vi "Updater Version Check.vi"(8 "에러 입력":errorcluster caption="에러 입력(에러 없음)") -> (0 "에러 출력":errorcluster, 1 "서버버전":string, 3 "업데이트?":bool)   [LabVIEW 2020]
uses:
  Support/Controls/Cmd_File path.ctl
  Support/Controls/Cmd_File Type.ctl
  Support/Controls/Cmd_Read Query.ctl
  Support/Public/Polymorph/ini Ctrl_Str.vi
  <vilib>/Utility/config.llb/Read Key (String).vi
  <vilib>/Utility/config.llb/NI_LVConfig.lvlib
  <vilib>/addons/database/NI_Database_API.lvlib
panel:
  out "로컬버전":string caption="값"
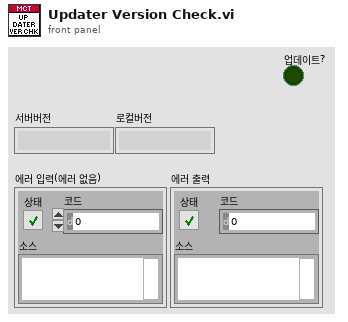
[diagram p1: front panel]
types:
  T1 = typedef "Cmd_Read Query.ctl" = enum16{"교정자 이름 얻기", "인증교정자 얻기", "기술책임자 얻기", "기책부책 얻기", "등록번호 얻기", "등록정보 얻기", "업체정보 얻기", "교정일자(CAMAS) 얻기", "교정일자(CALSTD) 얻기", "교정환경 얻기", "교정절차서 목록 얻기", "교정절차서명 얻기", "교정절차 목록얻기", "교정절차 얻기", "PROC 교정절차 얻기", "PROC SPEC 얻기", "교정절차(Func별) 얻기", "교정절차(Func_ext별) 얻기", "기관코드 얻기", "교정기능(세부분류) 얻기", "교정기능(모델) 얻기", "교정기능 목록 얻기", "교정기능 명칭 얻기", "교정기능 항목명칭 얻기", "DB (사용기준기) 얻기", "DB (기준기이름) 얻기", "DB (기준기이름목록) 얻기", "DB (기준기목록) 얻기", "DB (기준기값) 얻기", "DB (CMC) 얻기", "DB (FUNC) 얻기", "DB (CALNAME) 얻기", "DB (STDNAME) 얻기", "DB (SPEC) 얻기", "모델(항목전체) 얻기", "모델(최대범위) 얻기", "모델(최소범위) 얻기", "모델(최대최소) 얻기", "모델(범위조건) 얻기", "모델(등록요청) 얻기", "모델(형식별) 얻기", "모델(조건별) 얻기", "모델(모델검색) 얻기", "세부분류 목록 얻기", "기준기등록리스트 얻기", "STD Cal Date Check", "DB등록일자 얻기", "적용항목 얻기", "기타정보 얻기", "기준기요청 얻기", "서버버전 얻기"}
  T2 = typedef "Cmd_File Type.ctl" = enum16{"엑셀", "엑셀(2003)", "텍스트", "설정", "2진", "VI", "CSV", "LOG", "폴더"}
  T3 = typedef "Cmd_File path.ctl" = enum16{"에러로그", "데이터파일경로", "성적서원본", "지난성적서", "Data Files", "경로생성", "Updater", "Template", "설정파일경로", "FTP Upload", "Update 경로", "어플리케이션"}
  T4 = typedef "NI_Database_API.lvlib/Conn ObjectReference.ctl" = refnum<k1>
  T5 = typedef "NI_LVConfig.lvlib/Config Data RefNum.ctl" = refnum<k1>
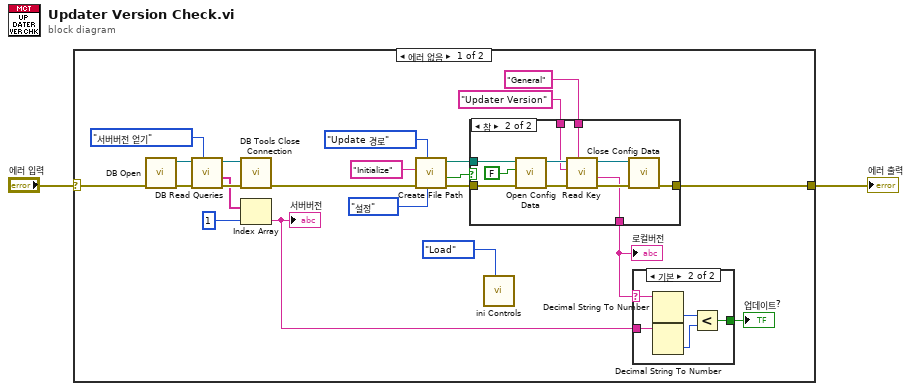
[diagram p0: block diagram]
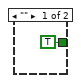
[diagram p2: hidden frame]
diagram:
  n1 = case shown="에러 없음" "에러 입력" {
    selector: "에러 입력" -> [w21 w43]
    tunnel: [w4 w43] -> w2
    frame No Error {
      n2 = call "DB Open.vi"("에러 입력"=w21) -> ("에러 출력"=w10:errorcluster, "참조 번호 출력"=w11:T4)  [unwired: 9 in]
      n3 = call "DB Read Queries.vi"("Query Command"=Cmd_Read_Query."서버버전 얻기", "에러 입력(에러 없음)"=w10, "참조 번호 입력"=w11) -> ("에러 출력"=w8:errorcluster, "Data (0번행)"=w6:string[], "참조 번호 출력"=w9:T4)  [unwired: 4 in, 2 out]
      n4 = call <vilib>:"DB Tools Close Connection.vi"("error in (no error)"=w8, "connection reference"=w9) -> ("error out"=w20:errorcluster)  [unwired: 5 in]
      n5 = Index Array(array=w6, index=1 ("비활성화된 인덱스 (열)")) -> (element=w14:string)
      "서버버전" <- w14
      n6 = call "Create File Path.vi"("파일타입"=Cmd_File_Type."설정", "항목"=Cmd_File_path."Update 경로", "에러 입력"=w20, "문자열 in"="Initialize" ("이름 또는 상대 경로")) -> ("error out"=w19:errorcluster, "파일존재?"=w15:bool, "파일경로"=w18:path)  [unwired: 4 in, 1 out]
      n7 = case shown="참" w15 {
        tunnel: w19 -> [w31 w42]
        tunnel: w18 -> [_ w41]
        tunnel: "General" ("section") -> [_ w38]
        tunnel: "Updater Version" ("key") -> [_ w37]
        tunnel: [w31 w34] -> w4
        tunnel: [_ w33] -> w13
        frame False {
        }
        frame True {
          n8 = call <vilib>:"Open Config Data.vi"("error in (no error)"=w42, "create file if necessary (T)"=FALSE, "configuration file path"=w41) -> ("error out"=w40:errorcluster, "refnum"=w39:T5)  [unwired: 6 in, 1 out]
          n9 = call-poly <vilib>:"Read Key.vi"("section"=w38, "error in (no error)"=w40, "key"=w37, "refnum"=w39) -> ("error out"=w36:errorcluster, "value"=w33:string, "refnum out"=w35:T5)  [unwired: 4 in, 1 out]
          n10 = call <vilib>:"Close Config Data.vi"("error in (no error)"=w36, "refnum"=w35) -> ("error out"=w34:errorcluster)  [unwired: 8 in, 1 out]
        }
      }
      "로컬버전" <- w13
      n11 = call-poly "ini Controls.vi"("Select"=enum16{"Save", "Load"}."Load") -> ()  [unwired: 8 in, 3 out]
      n12 = case shown="기본" w13 {
        selector: w13 -> [_ w26]
        tunnel: w14 -> [_ w30]
        tunnel: [TRUE w27] -> w12
        frame "" {
        }
        frame Default {
          n13 = Decimal String To Number(string=w26) -> (number=w28:i32)  [unwired: 2 in, 1 out]
          n14 = Decimal String To Number(string=w30) -> (number=w29:i32)  [unwired: 2 in, 1 out]
          n15 = Less?(x=w28, y=w29) -> (x < y?=w27:bool)
        }
      }
      "업데이트?" <- w12
    }
    frame Error {
    }
  }
  "에러 출력" <- w2
